vi "Basic.vi"() -> ()   [LabVIEW 2020]
uses:
  <vilib>/Utility/miscctls.llb/LVBoundsTypeDef.ctl
panel:
  in  "Boolean":bool
  out "Numeric Text.Text Colors:BG Color":u32(colorbox)
  out "Label.Text":string
  out "Bounds":T1
  in  "Number":dbl
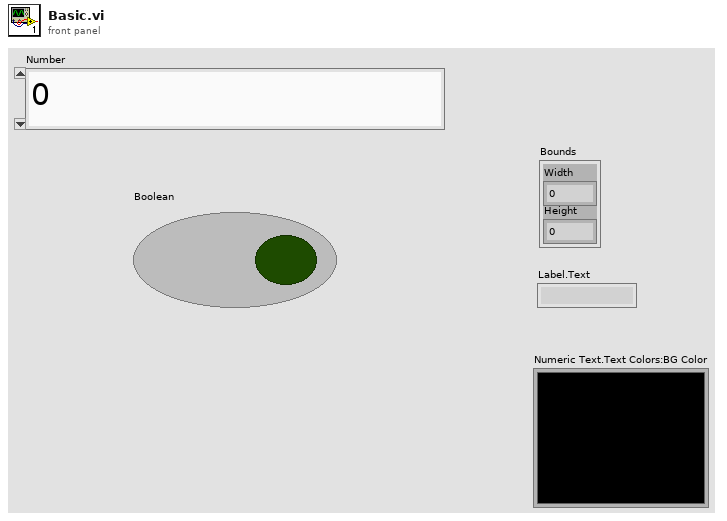
[diagram p1: front panel]
types:
  T1 = typedef "LVBoundsTypeDef.ctl" = cluster{"Width":u32, "Height":u32}
  T2 = enum8{"Enabled", "Disabled", "Disabled and Grayed Out"}
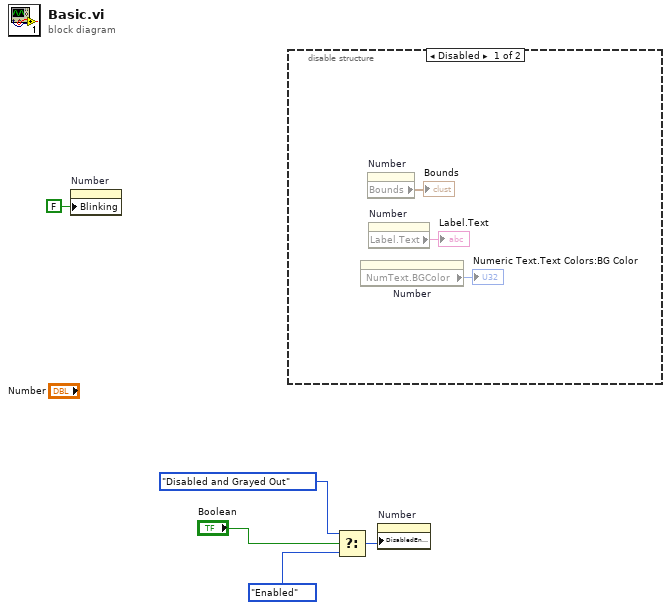
[diagram p0: block diagram]
diagram:
  n1 = property on="Number" class="DigNum (strict)"("Blinking"=FALSE) -> ()  [unwired: 2 in, 2 out]
  n2 = disable-structure shown="Disabled" {
    frame Disabled {
      n3 = property on="Number" class="DigNum (strict)"() -> ("NumText.BGColor"=→"Numeric Text.Text Colors:BG Color":u32)  [unwired: 2 in, 2 out]
      n4 = property on="Number" class="DigNum (strict)"() -> ("Bounds"=→"Bounds":T1)  [unwired: 2 in, 2 out]
      n5 = property on="Number" class="DigNum (strict)"() -> ("Label.Text"=→"Label.Text":string)  [unwired: 2 in, 2 out]
    }
    frame Enabled {
    }
  }
  n6 = Select(t=T2."Disabled and Grayed Out" ("Disabled"), s="Boolean", f=T2."Enabled" ("Disabled")) -> (s? t:f=w1:T2)
  n7 = property on="Number" class="DigNum (strict)"("DisabledEnum"=w1) -> ()  [unwired: 2 in, 2 out]
